vi "text.vi"() -> ()   [LabVIEW 2016]
uses:
  <vilib>/Simulation/Scripting/Companion Diagram/SimConfigNode/SimDog.xnode
  <vilib>/Simulation/Implementation/Shared/SIMSCR Execution Mode.ctl
  <vilib>/Simulation/Scripting/Companion Diagram/SimConfigNode/_simSolvers.ctl
  <vilib>/Simulation/Scripting/Companion Diagram/SimConfigNode/SimParams.ctl
  <vilib>/Simulation/Implementation/XNodeFramework/SimXNode/SimX.xnode
  <vilib>/Simulation/ContinuousLinear/Implementation/NILVSim Integrator new.llb/SIM Integrator (scalar).vi
  <vilib>/Simulation/SignalDisplay/Implementation/NILVSim Time Waveform.llb/SIM Time Waveform (scalar).vi
  <vilib>/Simulation/SignalDisplay/Implementation/NILVSim Buffer XY Graph.llb/SIM Buffer XY Graph (scalar).vi
  <vilib>/Simulation/ContinuousLinear/Implementation/NILVSim Transfer Function Direct.llb/SIM Transfer Function Direct (SISO).vi
  <vilib>/Simulation/SignalArithmetic/Implementation/NILVSim Gain.llb/SIM Gain (scalar).vi
  <vilib>/Simulation/Nonlinear/Implementation/NILVSim Switch.llb/SIM Switch (scalar).vi
  <vilib>/Simulation/Utility/Implementation/SIM Time.vi
  <vilib>/Analysis/baseanly.llb/Histogram.vi
  <vilib>/Analysis/NI_AALBase.lvlib
panel:
  out "2":T1(graph)
  out "3":T1(graph)
  out "4":T1(graph)
  out "size(s)":i32
  in  "Text":string="ABCDEFGHIJKLMNOPRSTUVYZ\n\na b c d e f g h i j k l m n o p r s t u v y z\n\n1 2 3 4 5 6 7 8 9 0\n\n+ - * =  /  < > .  ,  ;  : '' ! ? æ ~\"é \n\n@ £  #  $  ½  %  &  /  ( )  [ ] { } \n\n\n\n"
  out "?":string
  out "?":string
  out "?":string
  out "e3":waveform(dbl)(graph)
  out "e2":waveform(dbl)(graph)
  out "e1":waveform(dbl)(graph)
  out "X m":waveform(dbl)(graph)
  out "Y  m":waveform(dbl)(graph)
  out "YZ m":cluster{dbl, dbl}[](graph)
  out "XY m":cluster{dbl, dbl}[](graph)
  out "XZ m":cluster{dbl, dbl}[](graph)
  out "Z  m":waveform(dbl)(graph)
  out "XYs":cluster{dbl, dbl}[](graph)
  out "XZs":cluster{dbl, dbl}[](graph)
  out "YZs":cluster{dbl, dbl}[](graph)
  out "Zs":waveform(dbl)(graph)
  out "Ys":waveform(dbl)(graph)
  out "Xs":waveform(dbl)(graph)
  # "1234"
  # "orjinal"
  # "encrypted"
  # "decrypted"
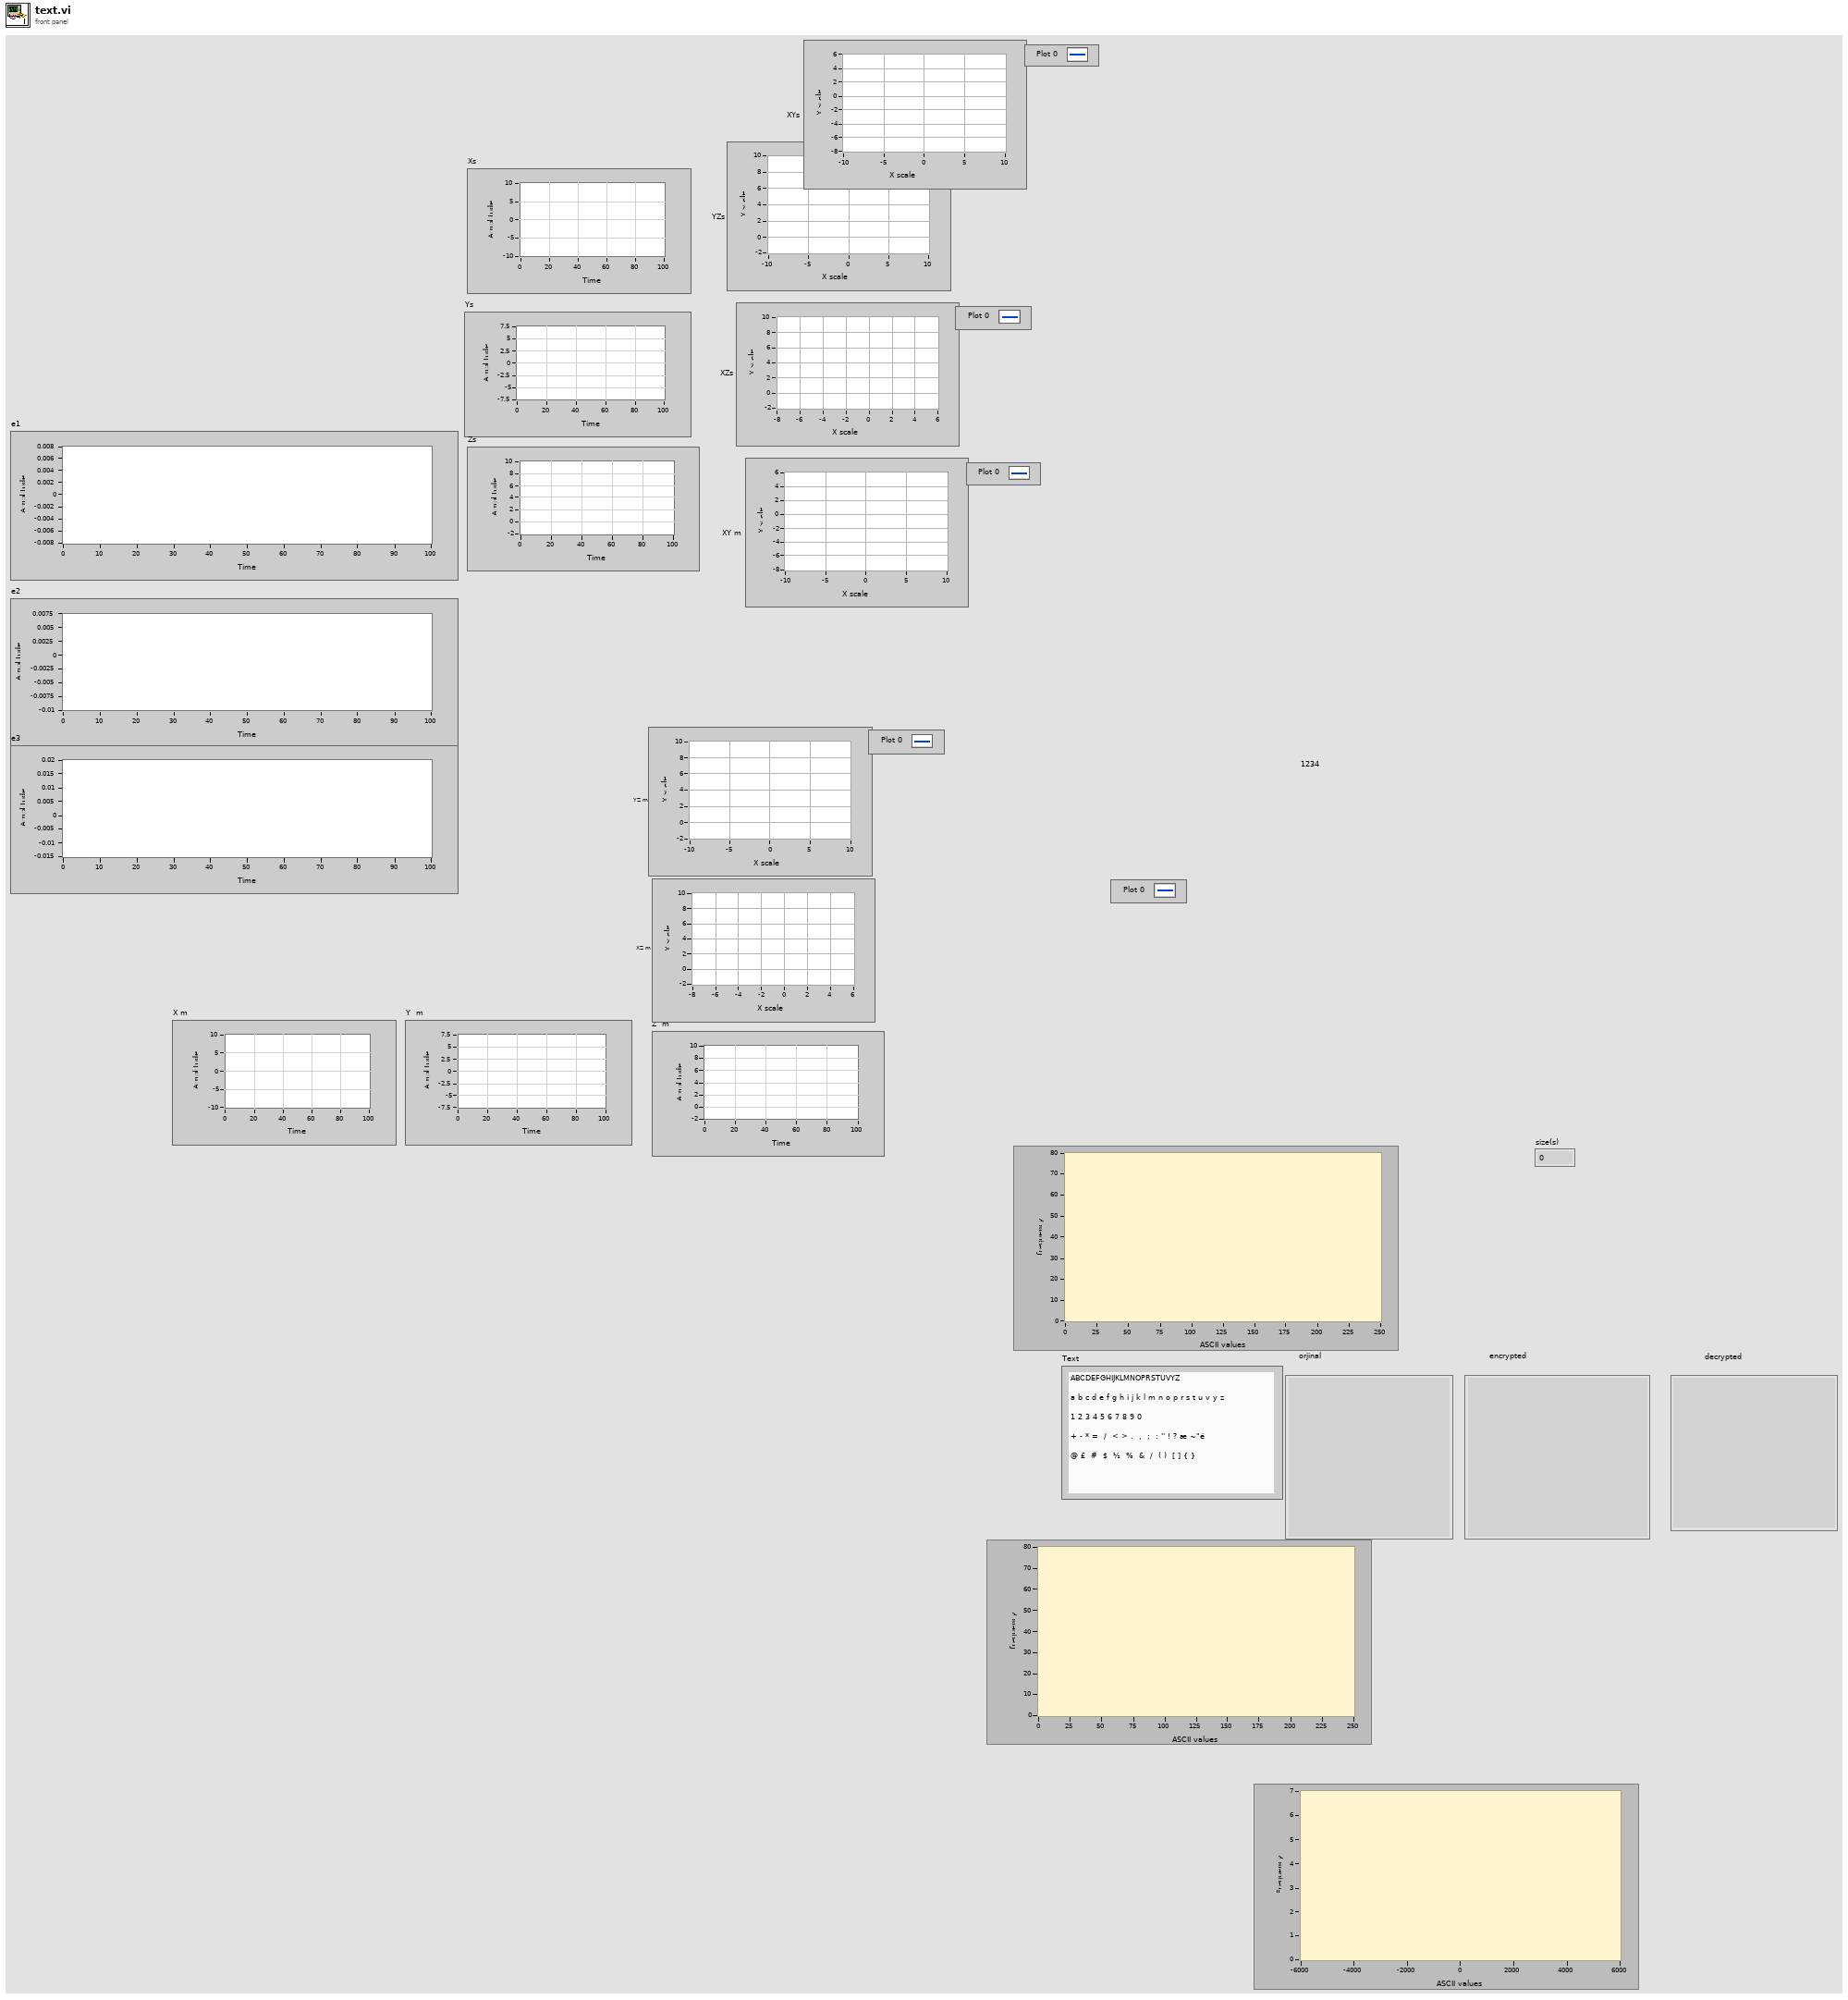
[diagram p1: front panel]
types:
  T1 = cluster{"X Values":dbl[], "Histogram: h(x)":i32[]}
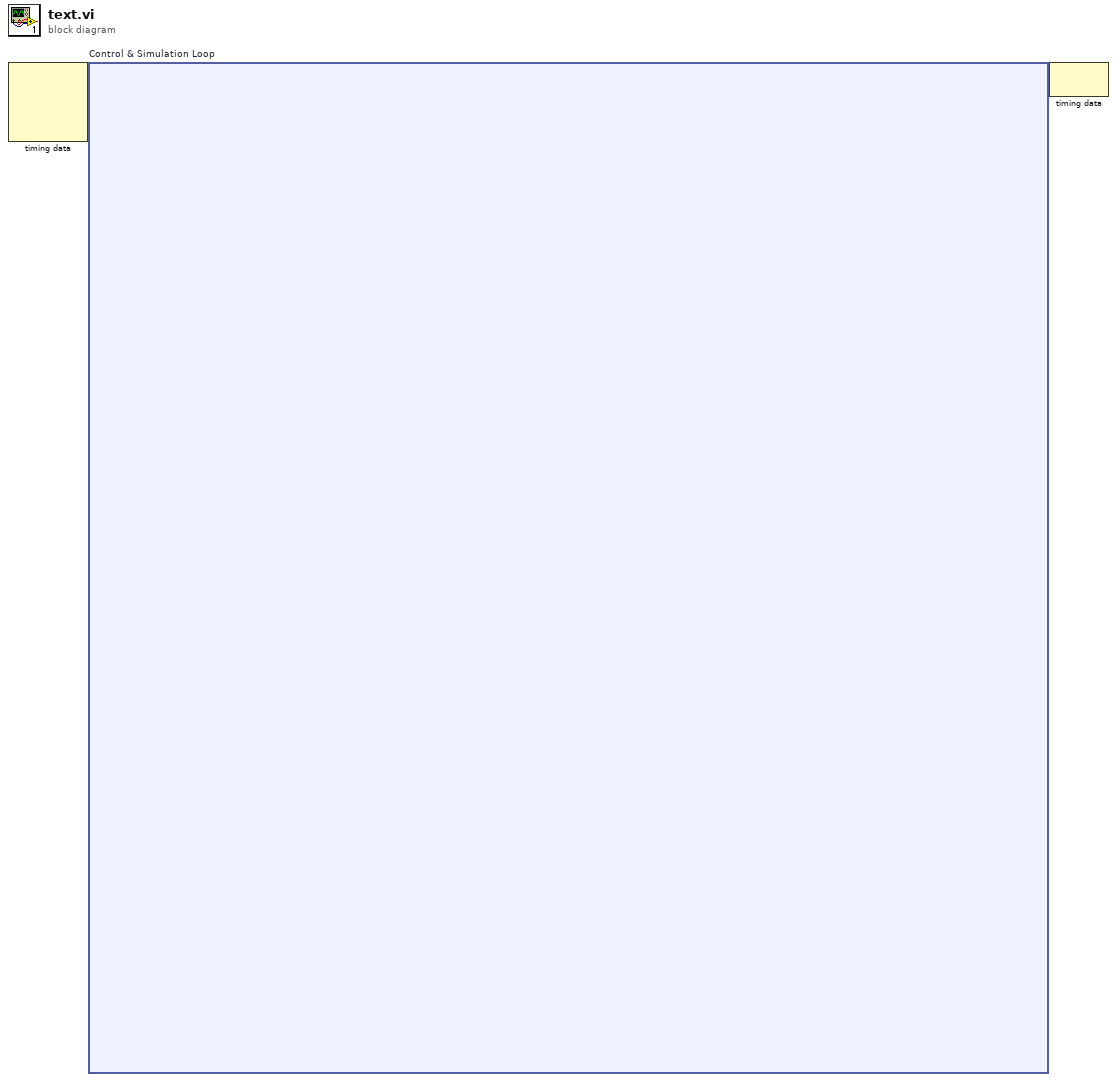
[diagram p0: block diagram]
diagram:
  n1 = node-c288() -> (w2:variant)  [unwired: 4 in]
  n2 = node-c254 "Control & Simulation Loop"(w2) -> (w1:variant)
  n3 = node-c288(w1) -> ()  [unwired: 1 out]
